vi "Write Ollama_URL.vi"(8 "error in (no error)":errorcluster, 10 "OpenAI_URL":string, 11 "llm_ollama_chatmodels in":refnum<class "llm_ollama_chatmodels.lvclass">) -> (0 "error out":errorcluster, 3 "llm_ollama_chatmodels out":refnum<class "llm_ollama_chatmodels.lvclass">)   [LabVIEW 2020, in "llm_ollama_chatmodels.lvclass"]
uses:
  llm_ollama_chatmodels.lvclass
  llm_ollama_chatmodels.lvclass/llm_ollama_chatmodels.ctl
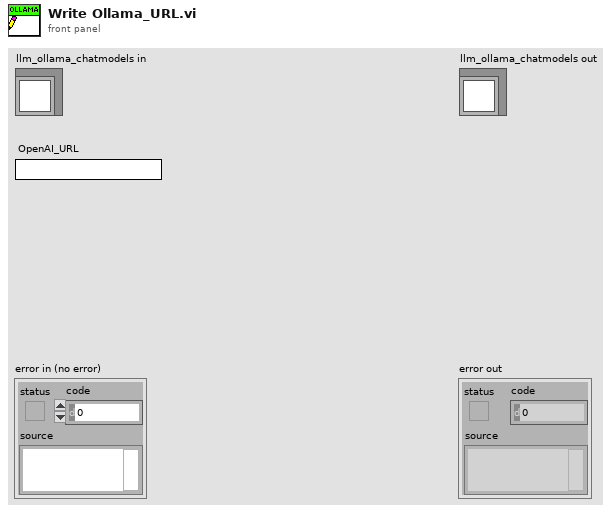
[diagram p1: front panel]
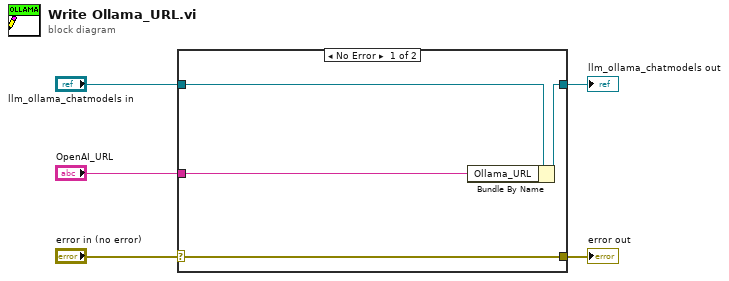
[diagram p0: block diagram]
diagram:
  n1 = case shown="No Error" "error in (no error)" {
    selector: "error in (no error)" -> [w9 w10]
    tunnel: [w9 w10] -> w4
    tunnel: [w7 w11] -> w2
    tunnel: "llm_ollama_chatmodels in" -> [w8 w11]
    tunnel: "OpenAI_URL" -> [w6 _]
    frame No Error {
      n2 = Bundle By Name(cluster=w8, "Ollama_URL"=w6) -> (w7:refnum<class "llm_ollama_chatmodels.lvclass">)
    }
    frame Error {
    }
  }
  "error out" <- w4
  "llm_ollama_chatmodels out" <- w2
